vi "ASI tester.vi"() -> ()   [LabVIEW 2015]
panel:
  out "Numeric":dbl
  in  "LOCK":bool
  in  "VISA resource in":refnum<visa-resource-name>="COM17"
  # "UNLOCK"
  # "Focus tester"
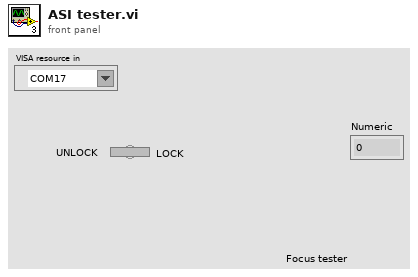
[diagram p1: front panel]
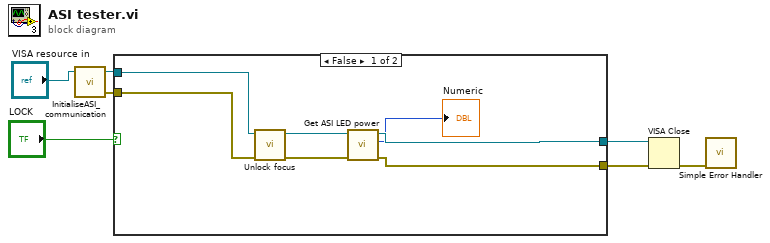
[diagram p0: block diagram]
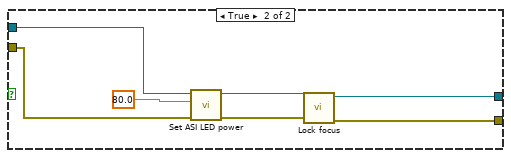
[diagram p2: hidden frame]
diagram:
  n1 = call "InitialiseASI_communication.vi"("COM port"="VISA resource in") -> ("error out"=w3:errorcluster, "VISA resource name out"=w1:refnum<visa-resource-name>)  [unwired: 3 in]
  n2 = case shown="False" "LOCK" {
    tunnel: w1 -> [w14 w17]
    tunnel: [w9 w19] -> w5
    tunnel: [w11 w18] -> w4
    tunnel: w3 -> [w13 w16]
    frame False {
      n3 = call "Unlock focus.vi"("error in"=w13, "VISA resource in"=w14) -> ("error out"=w10:errorcluster, "VISA resource out"=w12:refnum<visa-resource-name>)  [unwired: 8 in]
      n4 = call "Get ASI LED power.vi"("error in"=w10, "VISA resource in"=w12) -> ("error out"=w9:errorcluster, "LED power"=→"Numeric":i32, "VISA resource name out"=w11:refnum<visa-resource-name>)  [unwired: 7 in]
    }
    frame True {
      n5 = call "Set ASI LED power.vi"("error in"=w16, "New LED power"=80.0, "VISA resource in"=w17) -> ("error out"=w20:errorcluster, "VISA resource name out"=w21:refnum<visa-resource-name>)  [unwired: 7 in]
      n6 = call "Lock focus.vi"("error in"=w20, "VISA resource in"=w21) -> ("error out"=w19:errorcluster, "VISA resource out"=w18:refnum<visa-resource-name>)  [unwired: 8 in]
    }
  }
  n7 = VISA Close(VISA resource name=w4, error in (no error)=w5) -> (error out=w6:errorcluster)
  n8 = call <vilib>:"Simple Error Handler.vi"("error in (no error)"=w6) -> ()  [unwired: 4 in, 5 out]
